vi "Force Open New Log File Instance.vi"(8 "error in (no error)":errorcluster, 11 "Segmented Log in":refnum<class "Segmented Log.lvclass">) -> (0 "error out":errorcluster, 2 "Log Active":bool, 3 "Segmented Log out":refnum<class "Segmented Log.lvclass">)   [LabVIEW 2012, in "Waveform Data Logger Engine.lvlib" / "Segmented Log.lvclass"]
doc: "Forces the opening of a new log file instance if the configuration is still active. This first closes the current log file instance."
uses:
  Segmented Log.lvclass
  Segmented Log.lvclass/Segmented Log.ctl
  Shared/Classes/Log File Specifications/Log File Specification/Log File Specification.lvclass/Log File Specification.ctl
  Open Log File Instance.vi
  Shared/Classes/Log File Specifications/Log File Specification/Open Log File.vi
  Shared/Classes/Log File Specifications/Log File Specification/Set Path Tag.vi
  On File Open.vi
  Shared/Classes/Log File Specifications/Log File Specification/Set Filename Offset.vi
  Shared/Classes/Log File Specifications/Log File Specification/Build File Path.vi
  Shared/Classes/Log File Specifications/Log File Specification/Resolve File Conflicts.vi
  Shared/Classes/Log File Specifications/Log File Specification/Initialize Log File.vi
  <vilib>/Utility/libraryn.llb/Check if File or Folder Exists.vi
  <vilib>/Utility/error.llb/Error Cluster From Error Code.vi
  <vilib>/Utility/libraryn.llb/Get File Extension.vi
  <vilib>/Utility/libraryn.llb/Create Directory Recursive.vi
  Log Files/Log File/Log File.lvclass
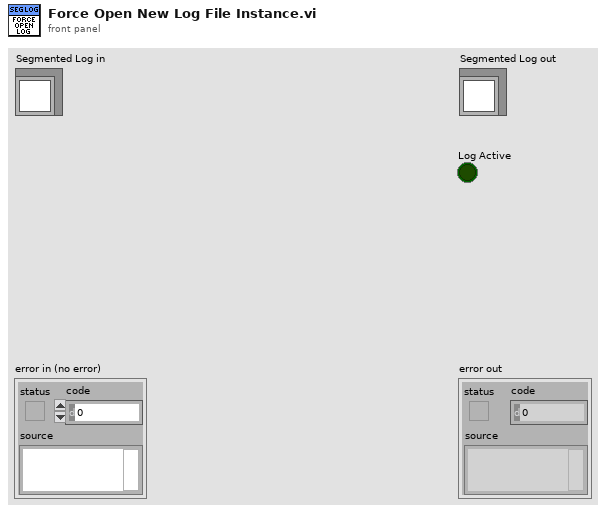
[diagram p1: front panel]
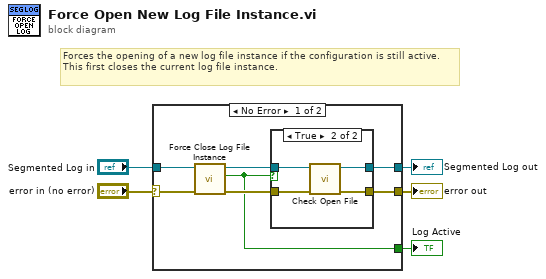
[diagram p0: block diagram]
diagram:
  # "Forces the opening of a new log file instance if the configuration is still active. This first closes the current log file instance."
  n1 = case shown="No Error" "error in (no error)" {
    selector: "error in (no error)" -> [w12 w20]
    tunnel: [w7 w20] -> w4
    tunnel: [w8 w19] -> w2
    tunnel: "Segmented Log in" -> [w11 w19]
    tunnel: [w6 _] -> w1
    frame No Error {
      n2 = call "Force Close Log File Instance.vi"("error in (no error)"=w12, "Segmented Log in"=w11) -> ("error out"=w10:errorcluster, "Log Active"=w6:bool, "Segmented Log out"=w9:refnum<class "Segmented Log.lvclass">)  [unwired: 7 in]
      n3 = case shown="True" w6 {
        tunnel: w10 -> [w13 w18]
        tunnel: w9 -> [w14 w17]
        tunnel: [w14 w16] -> w8
        tunnel: [w13 w15] -> w7
        frame False {
        }
        frame True {
          n4 = call "Check Open File.vi"("error in (no error)"=w18, "Segmented Log in"=w17) -> ("error out"=w15:errorcluster, "Segmented Log out"=w16:refnum<class "Segmented Log.lvclass">)  [unwired: 8 in]
        }
      }
    }
    frame Error {
    }
  }
  "error out" <- w4
  "Segmented Log out" <- w2
  "Log Active" <- w1
